vi "Get_Dest_Data.vi"(8 "error in (no error)":errorcluster, 11 "Class in":refnum<class "AB_Destination.lvclass">) -> (0 "error out":errorcluster, 2 "destName":T1, 3 "Class out":refnum<class "AB_Destination.lvclass">)   [LabVIEW 2020, in "AB_Destination.lvclass"]
uses:
  <vilib>/AppBuilder/AB_Classes/Destination/AB_Destination.lvclass
  <vilib>/AppBuilder/AB_Classes/Destination/AB_Destination.ctl
  <vilib>/AppBuilder/AB_Classes/Destination/AB_Destination.lvclass/AB_Destination.ctl
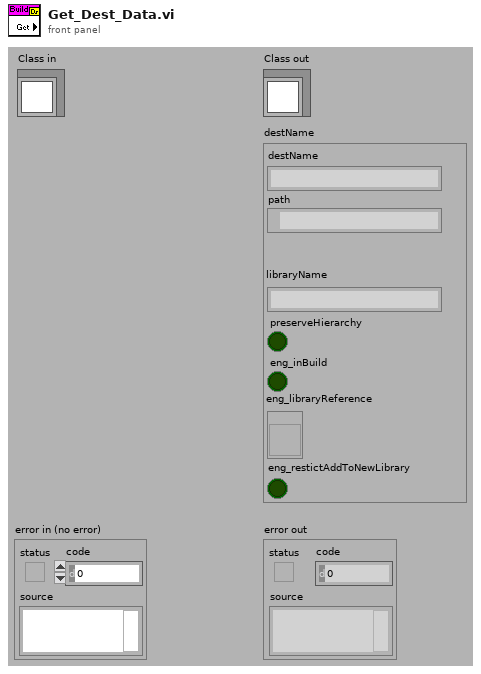
[diagram p1: front panel]
types:
  T1 = typedef "AB_Destination.ctl" = cluster{"destName":string, "path":path, "libraryName":string, "preserveHierarchy":bool, "eng_inBuild":bool, "eng_libraryReference":refnum<vi>, "eng_restictAddToNewLibrary":bool}
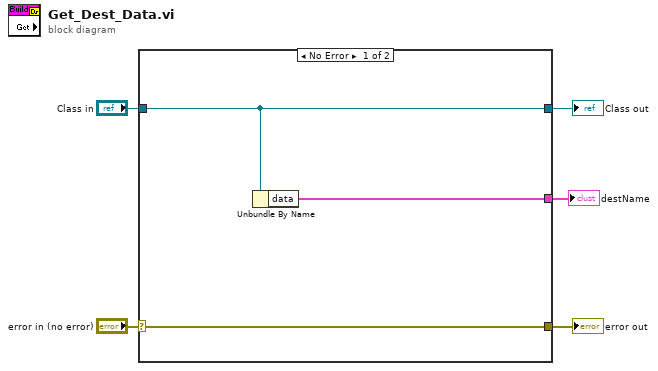
[diagram p0: block diagram]
diagram:
  n1 = case "Case" shown="No Error" "error in (no error)" {
    selector: "error in (no error)" -> [w8 w10]
    tunnel: [w8 w10] -> w4
    tunnel: [w7 w9] -> w2
    tunnel: "Class in" -> [w7 w9]
    tunnel: [w6 _] -> w1
    frame No Error {
      n2 = Unbundle By Name(w7) -> ("data"=w6:T1)
    }
    frame Error {
    }
  }
  "error out" <- w4
  "Class out" <- w2
  "destName" <- w1
